vi "KV_VolHead_Addr_Set.vi"(9 "设置的新地址":u8=1 min=1 max=10 step=1, 10 "原来地址":u8=1 min=1 max=10 step=1, 11 "MyIndex":u8) -> (3 "OK?":bool)   [LabVIEW 2015]
uses:
  <vilib>/Instr/_visa.llb/VISA Configure Serial Port (Instr).vi
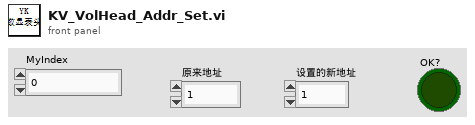
[diagram p1: front panel]
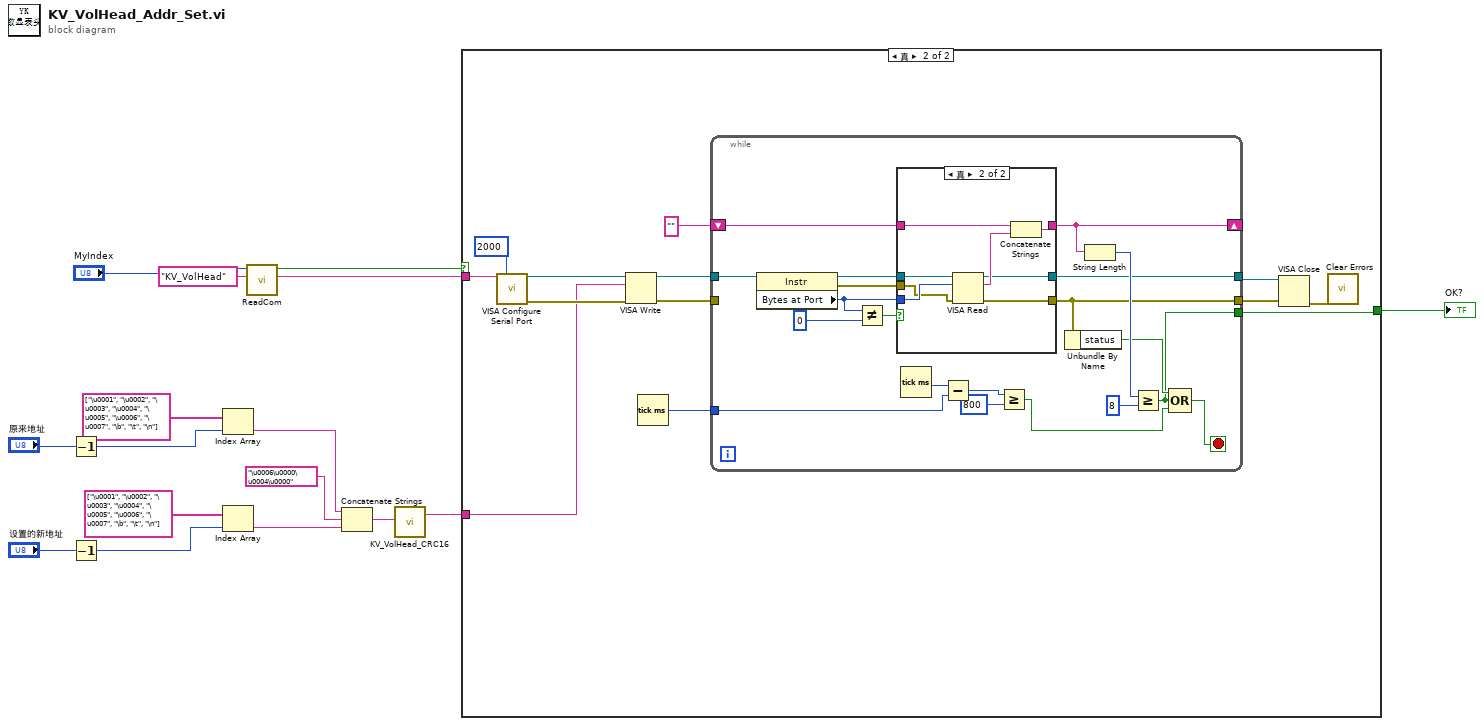
[diagram p0: block diagram]
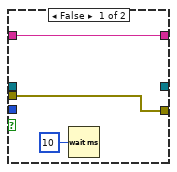
[diagram p3: hidden frame]
diagram:
  n1 = Decrement(x="原来地址") -> (x-1=w7:u8)
  n2 = Decrement(x="设置的新地址") -> (x-1=w6:u8)
  n3 = Index Array(array=string[] ["\u0001", "\u0002", "\u0003", "\u0004", "\u0005", "\u0006", "\u0007", "\b", "\t", "\n"], index=w7) -> (element=w12:string)
  n4 = Index Array(array=string[] ["\u0001", "\u0002", "\u0003", "\u0004", "\u0005", "\u0006", "\u0007", "\b", "\t", "\n"], index=w6) -> (element=w10:string)
  n5 = call "ReadCom.vi"("仪器名称"="KV_VolHead", "MyIndex"="MyIndex") -> ("COM"=w1:string, "OK?"=w2:bool)  [unwired: 7 in, 1 out]
  n6 = Concatenate Strings(w12, "\u0006\u0000\u0004\u0000" ("字符串"), w10) -> (w9:string)
  n7 = call "KV_VolHead_CRC16.vi"("input String"=w9) -> ("InPut +CRC"=w8:string)  [unwired: 1 out]
  n8 = case shown="真" w2 {
    tunnel: w8 -> [_ w23]
    tunnel: [_ w22] -> w5
    tunnel: w1 -> [_ w21]
    frame False {
    }
    frame True {
      n9 = call-poly "VISA Configure Serial Port"("VISA resource name"=w21, "timeout (10sec)"=u32 2000) -> ("VISA resource name out"=w29:refnum<visa-resource-name>, "error out"=w28:errorcluster)  [unwired: 12 in]
      n10 = VISA Write(VISA resource name=w29, write buffer=w23, error in (no error)=w28) -> (VISA resource name out=w26:refnum<visa-resource-name>, error out=w27:errorcluster)  [unwired: 1 out]
      n11 = Tick Count (ms)() -> (millisecond timer value=w24:u32)
      n12 = while {
        tunnel: w27 -> [_]
        tunnel: w26 -> [w49]
        shift-right: [w42] -> _
        shift-left: "" -> [w43]
        tunnel: w24 -> [w36]
        tunnel: [w32] -> w22
        tunnel: [w31] -> w19
        tunnel: [w30] -> w18
        stop <- w39 stop-if-true
        n13 = property class="Instr"(reference=w49) -> (reference out=w46:refnum<visa-resource-name>, error out=w44:errorcluster, "Bytes at Port"=w45:u32)  [unwired: 1 in]
        n14 = Not Equal?(x=w45, y=u32 0) -> (x != y?=w47:bool)
        n15 = case shown="真" w47 {
          tunnel: w46 -> [_ w60]
          tunnel: w45 -> [_ w59]
          tunnel: w44 -> [w50 w58]
          tunnel: w43 -> [w51 w57]
          tunnel: [w51 w55] -> w42
          tunnel: [w50 w54] -> w30
          tunnel: [_ w53] -> w31
          frame False {
            n16 = Wait (ms)(milliseconds to wait=u32 10 ("等待时间（毫秒）")) -> ()  [unwired: 1 out]
          }
          frame True {
            n17 = VISA Read(VISA resource name=w60, byte count=w59, error in (no error)=w58) -> (VISA resource name out=w53:refnum<visa-resource-name>, read buffer=w56:string, error out=w54:errorcluster)  [unwired: 1 out]
            n18 = Concatenate Strings(w57, w56) -> (w55:string)
          }
        }
        n19 = Tick Count (ms)() -> (millisecond timer value=w37:u32)
        n20 = Subtract(x=w37, y=w36) -> (x-y=w35:u32)
        n21 = Greater Or Equal?(x=w35, y=u32 800) -> (x >= y?=w33:bool)
        n22 = Unbundle By Name(w30) -> ("status"=w38:bool)
        n23 = String Length(string=w42) -> (length=w41:i32)
        n24 = Greater Or Equal?(x=w41, y=8) -> (x >= y?=w32:bool)
        n25 = Compound Arithmetic op=OR ("复合运算")(w38, w32, w33) -> (w39:bool)
      }
      n26 = VISA Close(VISA resource name=w19, error in (no error)=w18) -> (error out=w17:errorcluster)
      n27 = call <vilib>:"Clear Errors.vi"("error in (no error)"=w17) -> ()  [unwired: 5 in, 2 out]
    }
  }
  "OK?" <- w5
